vi "Position.vi"(11 "Shift":dbl) -> (3 "Position":cluster{"X":dbl, "Y":dbl, "Zpen":dbl})   [LabVIEW 2017]
uses:
  Program Files/National Instruments/LabVIEW 2019/user.lib/HapticSTM/HapticSTM.lvlib
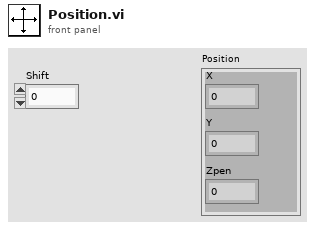
[diagram p1: front panel]
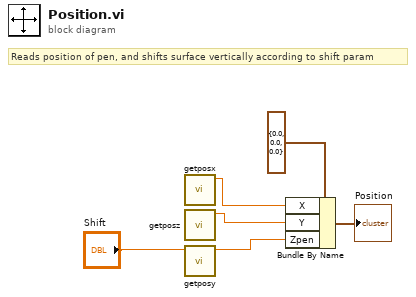
[diagram p0: block diagram]
diagram:
  # "Reads position of pen, and shifts surface vertically according to shift param"
  n1 = call "getposx.vi"() -> ("function return"=w2:dbl)  [unwired: 11 in]
  n2 = call "getposz.vi"() -> ("function return"=w3:dbl)  [unwired: 11 in]
  n3 = call "getposy.vi"("shift"="Shift") -> ("function return"=w1:dbl)  [unwired: 10 in]
  n4 = Bundle By Name(cluster=cluster{"X":dbl, "Y":dbl, "Zpen":dbl} {"X"=0.0, "Y"=0.0, "Zpen"=0.0} ("Position"), "X"=w2, "Y"=w3, "Zpen"=w1) -> (→"Position":cluster{"X":dbl, "Y":dbl, "Zpen":dbl})
